vi "USRP Generate Data.vi"(5 "Enum":enum16{"Sequential", "Pseudo Random"}(ring)) -> (6 "Data":u64)   [LabVIEW 2016]
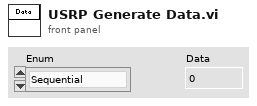
[diagram p1: front panel]
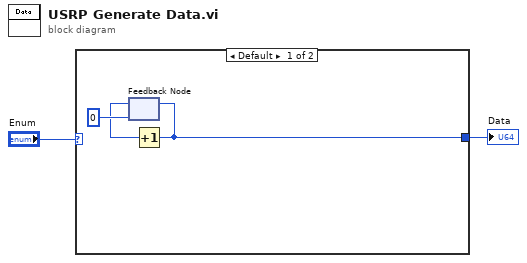
[diagram p0: block diagram]
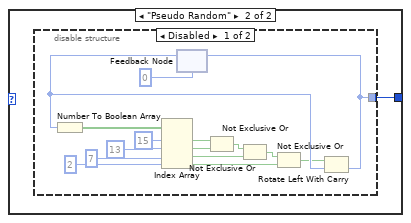
[diagram p2: hidden frame]
diagram:
  n1 = case shown="Default" "Enum" {
    tunnel: [w3 w6] -> w2
    frame Default {
      n2 = feedback #1(u64 0) -> (w4:u64)
      n3 = Increment(x=w4) -> (x+1=w3:u64)
      n4 = feedback-in #1(w3) -> ()
    }
    frame "Pseudo Random" {
      n5 = disable-structure shown="Disabled" {
        disable-tunnel: [w7 _] -> w6
        frame Disabled {
          n6 = feedback #2(u64 0) -> (w21:u64)
          n7 = Number To Boolean Array(number=w21) -> (Boolean array=w13:bool[])
          n8 = Index Array(array=w13, index #1=15 ("index"), index #2=13 ("index"), index #3=7 ("index"), index #4=2 ("index")) -> (element #1=w12:bool, element #2=w14:bool, element #3=w16:bool, element #4=w17:bool)
          n9 = Not Exclusive Or(1:w14, 2:w12) -> (0:w15:bool)
          n10 = Not Exclusive Or(1:w16, 2:w15) -> (0:w18:bool)
          n11 = Not Exclusive Or(1:w17, 2:w18) -> (0:w19:bool)
          n12 = Rotate Left With Carry(2:w21, 3:w19) -> (0:w7:u64)  [unwired: 1 out]
          n13 = feedback-in #2(w7) -> ()
        }
        frame Enabled {
        }
      }
    }
  }
  "Data" <- w2
